vi "UI Queue - FGV.vi"(7 "FGV States":T1, 8 "error in":errorcluster, 11 "VI In":refnum<vi>) -> (0 "error out":errorcluster, 3 "queue out":refnum<queue>)   [LabVIEW 2024, in "User Interface.lvlib"]
uses:
  Support/General Type Defs/FGV States.ctl
  Support/General Type Defs/Queue Message.ctl
  User Interface.lvlib
  Support/General Type Defs/General Type Defs.lvlib
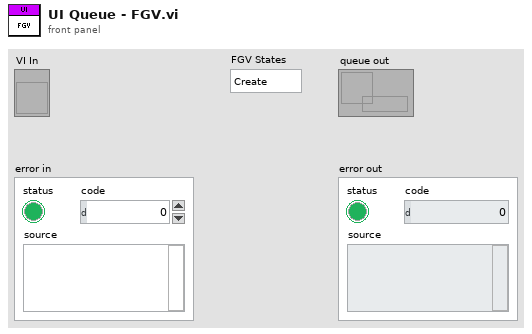
[diagram p1: front panel]
types:
  T1 = typedef "General Type Defs.lvlib/FGV States.ctl" = enum16{"Create", "Get", "Destroy"}
  T2 = typedef "General Type Defs.lvlib/Queue Message.ctl" = cluster{"Message":string, "Value":variant}
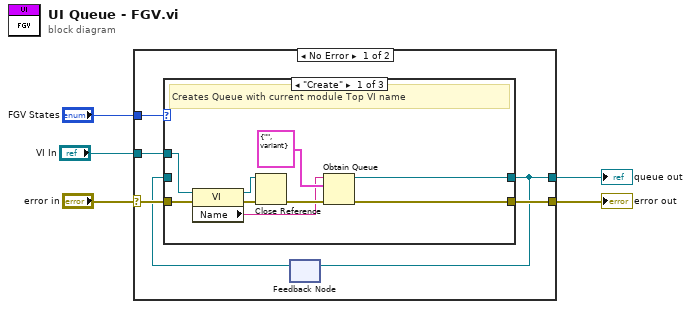
[diagram p0: block diagram]
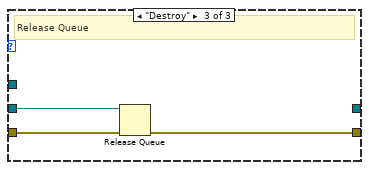
[diagram p3: hidden frame]
diagram:
  n1 = case shown="No Error" "error in" {
    selector: "error in" -> [w9 w26]
    tunnel: "FGV States" -> [w11 _]
    tunnel: [w10 w26] -> w4
    tunnel: [w8 _] -> w2
    tunnel: "VI In" -> [w6 _]
    frame No Error {
      n2 = feedback #1() -> (w7:refnum<queue>)  [unwired: 1 in]
      n3 = case shown="\"Create\"" w11 {
        tunnel: [w20 w21 w24] -> w10
        tunnel: w9 -> [w15 w21 w25]
        tunnel: [w18 w22 _] -> w8
        tunnel: w7 -> [_ w22 w23]
        tunnel: w6 -> [w13 _ _]
        frame "Create" {
          # "Creates Queue with current module Top VI name"
          n4 = property class="VI"(reference=w13, error in=w15) -> (reference out=w17:refnum<vi>, error out=w16:errorcluster, "Name"=w12:string)
          n5 = Close Reference(reference=w17, error in (no error)=w16) -> (error out=w14:errorcluster)
          n6 = Obtain Queue(name (unnamed)=w12, element data type=T2 {"Message"="", "Value"=variant}, error in (no error)=w14) -> (queue out=w18:refnum<queue>, error out=w20:errorcluster)  [unwired: 2 in, 1 out]
        }
        frame "Get", Default {
          # "Gets Queue"
        }
        frame "Destroy" {
          # "Release Queue"
          n7 = Release Queue(queue=w23, error in (no error)=w25) -> (error out=w24:errorcluster)  [unwired: 1 in, 2 out]
        }
      }
      n8 = feedback-in #1(w8) -> ()
    }
    frame Error {
    }
  }
  "error out" <- w4
  "queue out" <- w2
